vi "ws_cgi get raw file.vi"(7 "Content-type (\"application/octet-stream\")":string="application/octet-stream", 8 "error in (no error)":errorcluster, 9 "Filename (\"\")":string, 10 "Content (\"\")":string, 11 "httpRequestID":u32) -> (0 "error out":errorcluster, 2 "Packed Content":string)   [LabVIEW 2011]
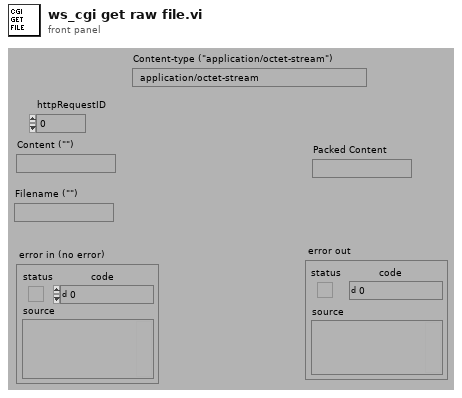
[diagram p1: front panel]
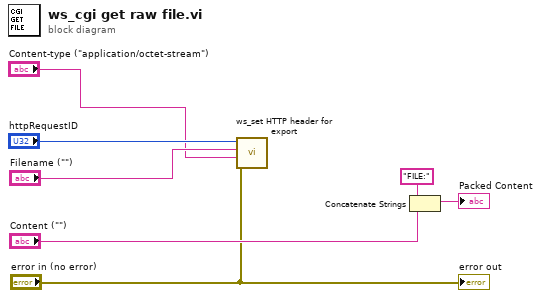
[diagram p0: block diagram]
diagram:
  n1 = call "ws_set HTTP header for export.vi"("error in (no error)"="error in (no error)", "Content-type (\"application/octet-stream\")"="Content-type (\"application/octet-stream\")", "filename (\"\")"="Filename (\"\")", "httpRequestID"="httpRequestID") -> ()  [unwired: 1 in, 7 out]
  n2 = Concatenate Strings("FILE:" ("Template (\"\")"), "Content (\"\")") -> (→"Packed Content":string)
  "error out" <- "error in (no error)"
